vi "Write address.vi"(5 "address":string="192.168.1.7", 9 "Downloader in":refnum<class "Downloader.lvclass">) -> (3 "Downloader out":refnum<class "Downloader.lvclass">)   [LabVIEW 2014, in "Downloader.lvclass"]
uses:
  Downloader.lvclass
  Downloader.lvclass/Downloader.ctl
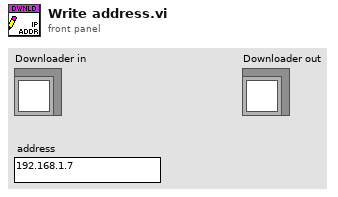
[diagram p1: front panel]
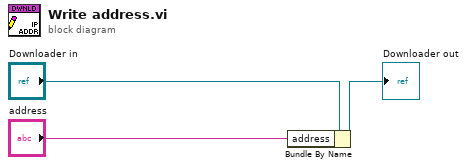
[diagram p0: block diagram]
diagram:
  n1 = Bundle By Name(cluster="Downloader in", "address"="address") -> (→"Downloader out":refnum<class "Downloader.lvclass">)
